vi "Дешифратор семисегментного индикатора.vi"(1 "X":T2) -> (0 "R":T1)   [LabVIEW 2013]
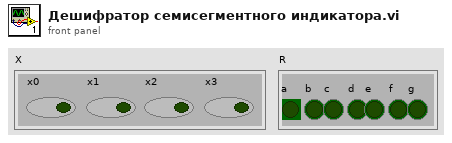
[diagram p1: front panel]
types:
  T1 = cluster{"a":bool, "b":bool, "c":bool, "d":bool, "e":bool, "f":bool, "g":bool}
  T2 = cluster{"x0":bool, "x1":bool, "x2":bool, "x3":bool}
  T3 = cluster{bool, bool, bool, bool, bool, bool, bool}
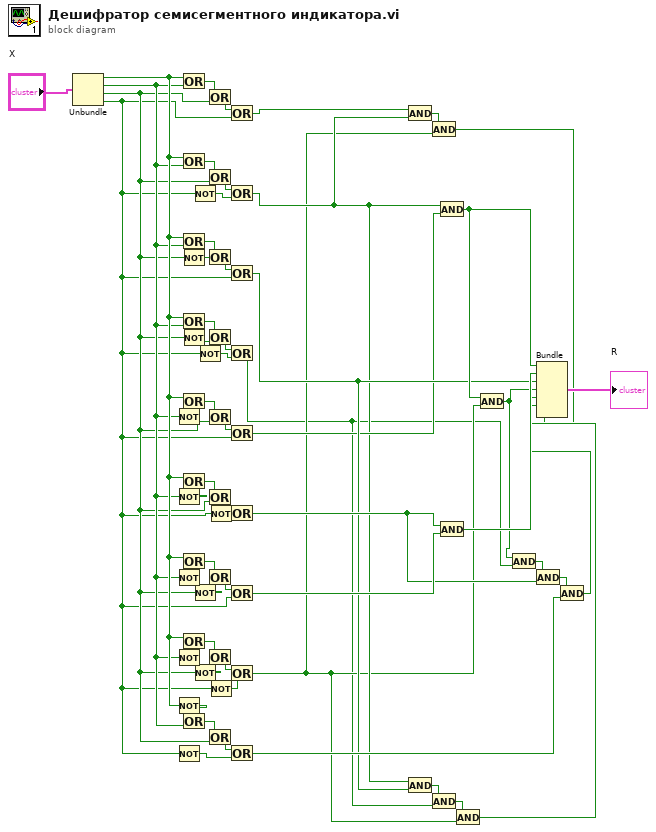
[diagram p0: block diagram]
diagram:
  n1 = Unbundle("X") -> ("x0"=w26:bool, "x1"=w25:bool, "x2"=w24:bool, "x3"=w1:bool)
  n2 = Not(x=w25) -> (.not. x?=w37:bool)
  n3 = Not(x=w25) -> (.not. x?=w36:bool)
  n4 = Not(x=w25) -> (.not. x?=w34:bool)
  n5 = Not(x=w25) -> (.not. x?=w32:bool)
  n6 = Not(x=w26) -> (.not. x?=w27:bool)
  n7 = Not(x=w1) -> (.not. x?=w2:bool)
  n8 = Or(x=w26, y=w25) -> (x .or. y?=w57:bool)
  n9 = Or(x=w26, y=w25) -> (x .or. y?=w55:bool)
  n10 = Or(x=w26, y=w25) -> (x .or. y?=w53:bool)
  n11 = Not(x=w24) -> (.not. x?=w40:bool)
  n12 = Or(x=w26, y=w25) -> (x .or. y?=w51:bool)
  n13 = Not(x=w24) -> (.not. x?=w38:bool)
  n14 = Or(x=w26, y=w37) -> (x .or. y?=w49:bool)
  n15 = Or(x=w26, y=w36) -> (x .or. y?=w47:bool)
  n16 = Or(x=w26, y=w34) -> (x .or. y?=w45:bool)
  n17 = Or(x=w26, y=w32) -> (x .or. y?=w43:bool)
  n18 = Or(x=w27, y=w25) -> (x .or. y?=w29:bool)
  n19 = Not(x=w1) -> (.not. x?=w41:bool)
  n20 = Not(x=w24) -> (.not. x?=w33:bool)
  n21 = Not(x=w24) -> (.not. x?=w31:bool)
  n22 = Not(x=w1) -> (.not. x?=w39:bool)
  n23 = Or(x=w57, y=w24) -> (x .or. y?=w56:bool)
  n24 = Or(x=w55, y=w24) -> (x .or. y?=w54:bool)
  n25 = Or(x=w53, y=w40) -> (x .or. y?=w52:bool)
  n26 = Or(x=w51, y=w38) -> (x .or. y?=w50:bool)
  n27 = Or(x=w49, y=w24) -> (x .or. y?=w48:bool)
  n28 = Or(x=w47, y=w24) -> (x .or. y?=w46:bool)
  n29 = Or(x=w45, y=w33) -> (x .or. y?=w44:bool)
  n30 = Or(x=w43, y=w31) -> (x .or. y?=w42:bool)
  n31 = Or(x=w29, y=w24) -> (x .or. y?=w28:bool)
  n32 = Not(x=w1) -> (.not. x?=w35:bool)
  n33 = Not(x=w1) -> (.not. x?=w30:bool)
  n34 = Or(x=w56, y=w1) -> (x .or. y?=w7:bool)
  n35 = Or(x=w54, y=w41) -> (x .or. y?=w6:bool)
  n36 = Or(x=w52, y=w1) -> (x .or. y?=w11:bool)
  n37 = Or(x=w50, y=w39) -> (x .or. y?=w3:bool)
  n38 = Or(x=w48, y=w1) -> (x .or. y?=w10:bool)
  n39 = Or(x=w46, y=w35) -> (x .or. y?=w17:bool)
  n40 = Or(x=w44, y=w1) -> (x .or. y?=w22:bool)
  n41 = Or(x=w42, y=w30) -> (x .or. y?=w5:bool)
  n42 = Or(x=w28, y=w2) -> (x .or. y?=w15:bool)
  n43 = And(x=w7, y=w6) -> (x .and. y?=w8:bool)
  n44 = And(x=w6, y=w11) -> (x .and. y?=w12:bool)
  n45 = And(x=w8, y=w5) -> (x .and. y?=w4:bool)
  n46 = And(x=w12, y=w3) -> (x .and. y?=w13:bool)
  n47 = And(x=w6, y=w10) -> (x .and. y?=w20:bool)
  n48 = And(x=w17, y=w22) -> (x .and. y?=w21:bool)
  n49 = And(x=w13, y=w5) -> (x .and. y?=w9:bool)
  n50 = And(x=w20, y=w5) -> (x .and. y?=w19:bool)
  n51 = And(x=w19, y=w3) -> (x .and. y?=w18:bool)
  n52 = And(x=w18, y=w17) -> (x .and. y?=w16:bool)
  n53 = And(x=w16, y=w15) -> (x .and. y?=w14:bool)
  n54 = Bundle(w20, w21, w11, w19, w14, w9, w4) -> (→"R":T3)  [unwired: 1 in]
